vi "Ortalama Hesaplama.vi"() -> ()   [LabVIEW 2014]
panel:
  out "Sonuç":string
  in  "Ortalama":dbl
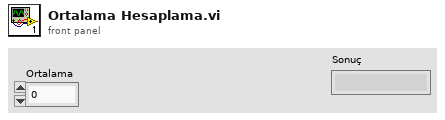
[diagram p1: front panel]
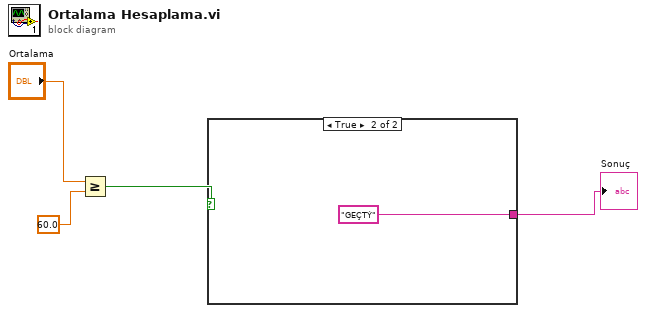
[diagram p0: block diagram]
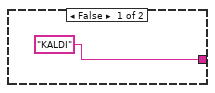
[diagram p2: hidden frame]
diagram:
  n1 = Greater Or Equal?(x="Ortalama", y=60.0) -> (x >= y?=w2:bool)
  n2 = case shown="True" w2 {
    tunnel: ["KALDI" "GEÇTÝ"] -> w3
    frame False {
    }
    frame True {
    }
  }
  "Sonuç" <- w3
